vi "Sine_Square_Tri.vi"() -> ()   [LabVIEW 2013]
uses:
  <vilib>/sound2/lvsound2.llb/Sampling Mode.ctl
  <vilib>/sound2/lvsound2.llb/Sound Data Format.ctl
  <vilib>/Analysis/4window.llb/windowTd.ctl
  <vilib>/measure/maspectr.llb/Power Spectrum and PSD Export Mode.ctl
  <vilib>/sound2/lvsound2.llb/Sound Output Set Volume (Single).vi
  <vilib>/measure/maspectr.llb/FFT Spectrum (Mag-Phase) for 1 Chan.vi
  <vilib>/measure/maspectr.llb/FFT Power Spectrum and PSD for 1 Chan.vi
  <vilib>/sound2/lvsound2.llb/Sound Output Write (DBL Single).vi
  <vilib>/measure/NI_MAPro.lvlib
  <vilib>/Analysis/NI_AALPro.lvlib
panel:
  out "Magnitude":cluster{"f0":dbl, "df":dbl, "magnitude":dbl[]}(graph)
  out "Power Spectral Density":cluster{"f0":dbl, "df":dbl, "magnitude":dbl[]}(graph)
  in  "Device ID":u32
  in  "Stop":bool
  in  "Frequency":dbl(knob)=500.0 scale=0.0..10000.0
  out "Generated Sound":waveform(dbl)(graph)
  in  "Volume":dbl(knob)=50.0 scale=0.0..100.0
  out "Y max":dbl format="%0.2f"
  out "Y min":dbl format="%0.2f"
  out "Hz":dbl
  out "Numeric":dbl
  in  "Phase":dbl(knob) scale=0.0..10.0
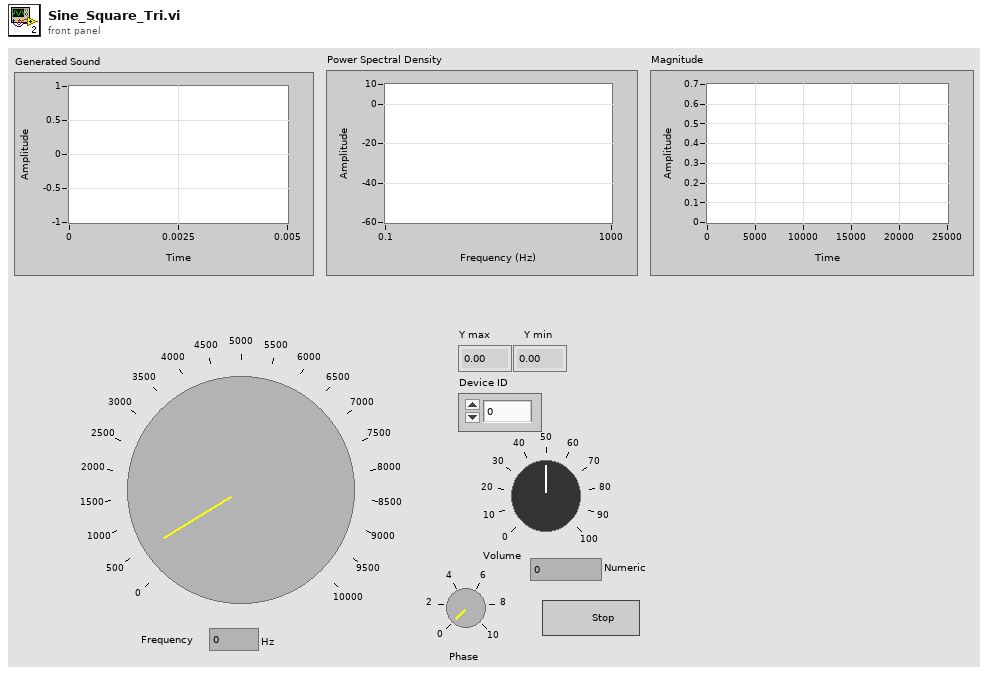
[diagram p1: front panel]
types:
  T1 = typedef "Sound Data Format.ctl" = cluster{"sample rate (S/s)":dbl, "number of channels":i32, "bits per sample":i32}
  T2 = typedef "Sampling Mode.ctl" = i32
  T3 = typedef "Sound Output Task ID.ctl" = u32
  T4 = cluster{"averaging mode":enum16{"No averaging", "Vector averaging", "RMS averaging", "Peak hold"}, "weighting mode":enum16{"Linear", "Exponential"}, "number of averages":u32}
  T5 = cluster{"dB On (F)":bool, "unwrap phase (F)":bool, "convert to degree (F)":bool}
  T6 = typedef "NI_AALPro.lvlib/windowTd.ctl" = u32
  T7 = typedef "NI_MAPro.lvlib/Power Spectrum and PSD Export Mode.ctl" = u16
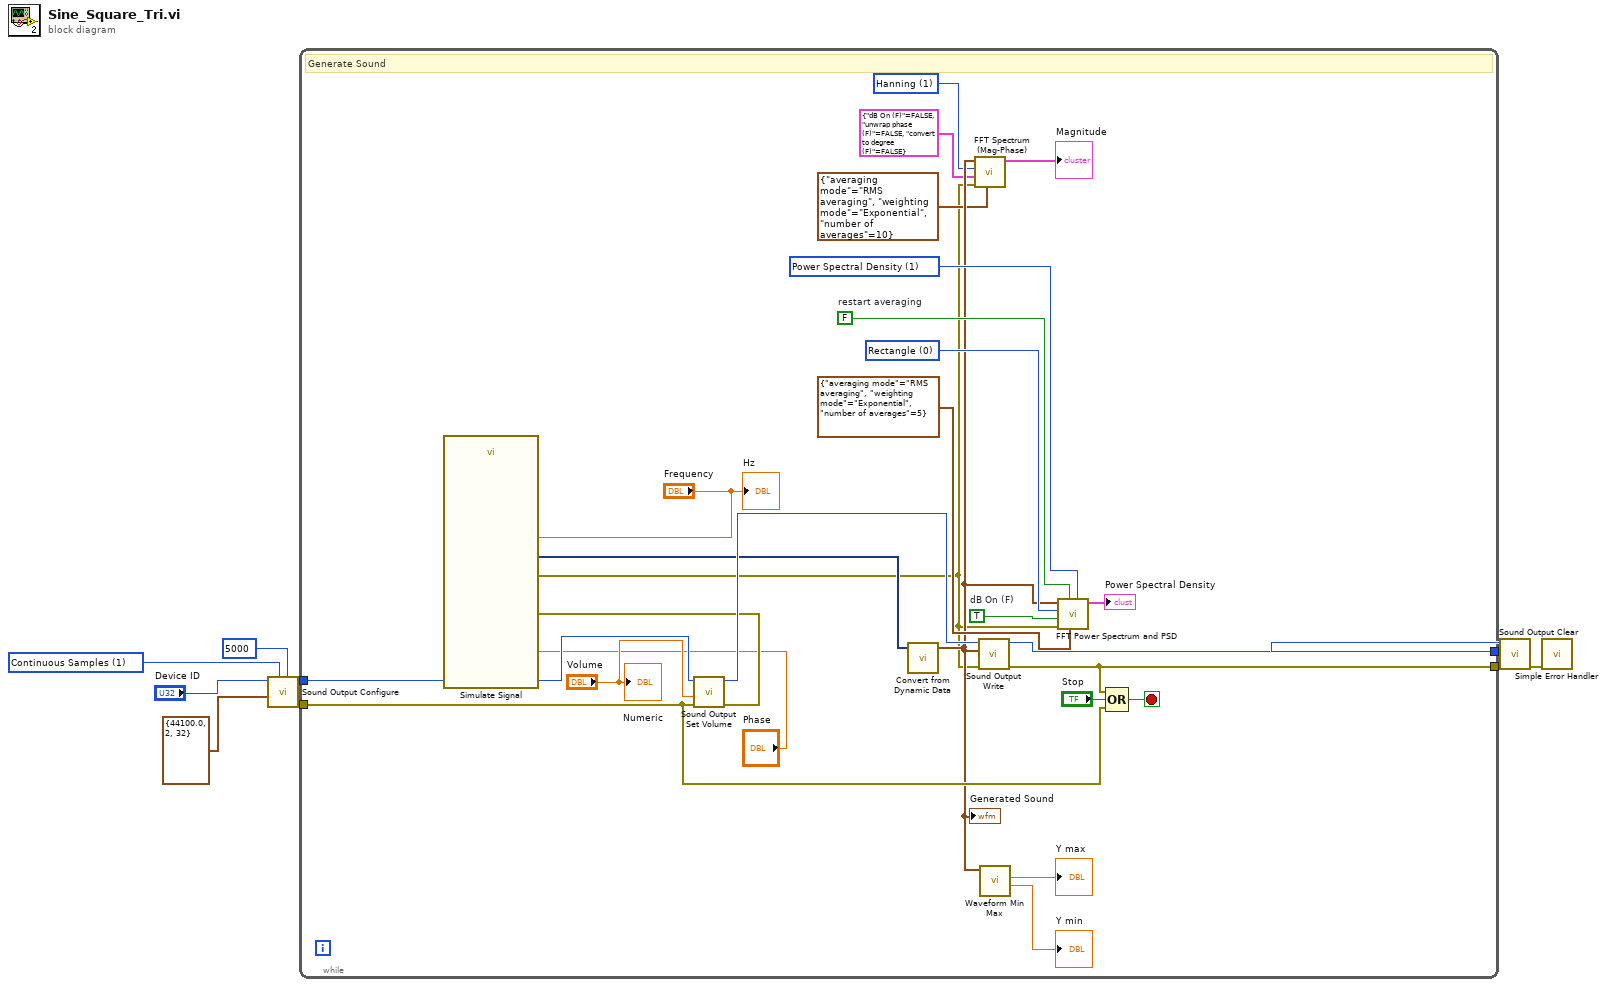
[diagram p0: block diagram]
diagram:
  w4 = T2 1 items=["Finite Samples", "Continuous Samples"] ("sample mode")
  n1 = call <vilib>:"Sound Output Configure.vi"("number of samples/ch"=5000 ("Number of Samples/ch"), "sample mode"=w4, "sound format"=T1 {"sample rate (S/s)"=44100.0, "number of channels"=2, "bits per sample"=32} ("Sound Format"), "device ID"="Device ID") -> ("error out"=w9:errorcluster, "task ID"=w8:T3)  [unwired: 6 in]
  n2 = while {
    tunnel: w8 -> [w33]
    tunnel: [w35] -> w6
    tunnel: w9 -> [w22]
    tunnel: [w25] -> w7
    stop <- w23 stop-if-true
    w14 = T6 1 items=["Rectangle"=0, "Hanning"=1, "Hamming"=2, "Blackman-Harris"=3, "Exact Blackman"=4, "Blackman"=5, "Flat Top"=6, "4 Term B-Harris "=7, "7 Term B-Harris"=8, "Low Sidelobe"=9, "Blackman Nuttall"=11, "Triangle"=30, "Bartlett-Hanning"=31, "Bohman"=32, "Parzen"=33, "Welch"=34, "Kaiser"=60, "Dolph-Chebyshev"=61, "Gaussian"=62] ("window")
    w21 = T7 1 items=["Power Spectrum", "Power Spectral Density"] ("export mode")
    w20 = T6 0 items=["Rectangle"=0, "Hanning"=1, "Hamming"=2, "Blackman-Harris"=3, "Exact Blackman"=4, "Blackman"=5, "Flat Top"=6, "4 Term B-Harris "=7, "7 Term B-Harris"=8, "Low Sidelobe"=9, "Blackman Nuttall"=11, "Triangle"=30, "Bartlett-Hanning"=31, "Bohman"=32, "Parzen"=33, "Welch"=34, "Kaiser"=60, "Dolph-Chebyshev"=61, "Gaussian"=62] ("window")
    w18 = FALSE  # restart averaging
    w19 = TRUE  # dB On (F)
    # "Generate Sound"
    n3 = call-poly <vilib>:"Sound Output Set Volume.vi"("error in (no error)"=w22, "volume"="Volume", "task ID"=w33) -> ("error out"=w32:errorcluster, "task ID out"=w34:T3)  [unwired: 7 in]
    n4 = call "Simulate Signal"("Frequency"="Frequency", "Phase"="Phase", "error in (no error)"=w32) -> ("Sine"=w31:dynamicdata, "error out"=w10:errorcluster)  [unwired: 11 in]
    n5 = call "Convert from Dynamic Data"("Dynamic Data Type"=w31) -> ("Waveform"=w15:waveform(dbl))  [unwired: 3 in]
    "Generated Sound" <- w15
    n6 = call-poly <vilib>:"FFT Spectrum (Mag-Phase).vi"("averaging parameters"=T4 {"averaging mode"=enum."RMS averaging", "weighting mode"=enum."Exponential", "number of averages"=10}, "error in (no error)"=w10, "view"=T5 {"dB On (F)"=FALSE, "unwrap phase (F)"=FALSE, "convert to degree (F)"=FALSE}, "window"=w14, "time signal"=w15) -> ("magnitude"=→"Magnitude":cluster{"f0":dbl, "df":dbl, "magnitude":dbl[]})  [unwired: 2 in, 4 out]
    n7 = call-poly <vilib>:"Sound Output Write.vi"("error in (no error)"=w10, "data"=w15, "task ID"=w34) -> ("error out"=w25:errorcluster, "task ID out"=w35:T3)  [unwired: 7 in]
    n8 = call <vilib>:"Waveform Min Max.vi"("waveform in"=w15) -> ("Y min"=→"Y min":dbl, "Y max"=→"Y max":dbl)  [unwired: 5 in, 4 out]
    n9 = call-poly <vilib>:"FFT Power Spectrum and PSD.vi"("export mode"=w21, "averaging parameters"=T4 {"averaging mode"=enum."RMS averaging", "weighting mode"=enum."Exponential", "number of averages"=5}, "restart averaging (F)"=w18, "error in (no error)"=w10, "dB On (F)"=w19, "window"=w20, "time signal"=w15) -> ("Power Spectrum / PSD"=→"Power Spectral Density":cluster{"f0":dbl, "df":dbl, "magnitude":dbl[]})  [unwired: 1 in, 3 out]
    n10 = Compound Arithmetic op=OR(w25, "Stop", w22) -> (w23:bool)
    "Hz" <- "Frequency"
    "Numeric" <- "Volume"
  }
  n11 = call <vilib>:"Sound Output Clear.vi"("error in (no error)"=w7, "task ID"=w6) -> ("error out"=w2:errorcluster)  [unwired: 9 in]
  n12 = call <vilib>:"Simple Error Handler.vi"("error in (no error)"=w2) -> ()  [unwired: 4 in, 5 out]
